vi "Migrate Shared Dependencies.vi"(0 "project path":path, 5 "measurement path":path, 7 "common dependencies":path[](array[path]), 11 "error in":errorcluster) -> (4 "outside items":string[](array[string]), 6 "library":T1[](array[typedef]), 15 "error out":errorcluster)   [LabVIEW 2021, in "Multiple Converter.lvlib"]
uses:
  Multiple Converter.lvlib
  TypeDefs/Library Info.ctl
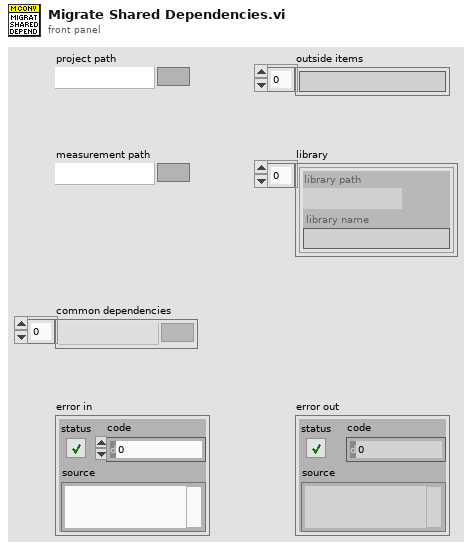
[diagram p1: front panel]
types:
  T1 = typedef "Multiple Converter.lvlib/Library Info.ctl" = cluster{"library path":path, "library name":string}
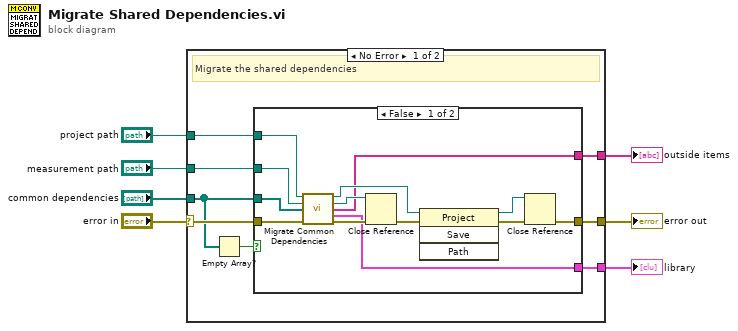
[diagram p0: block diagram]
diagram:
  n1 = case shown="No Error" "error in" {
    selector: "error in" -> [w14 w30]
    tunnel: [w15 w30] -> w7
    tunnel: "common dependencies" -> [w11 _]
    tunnel: "project path" -> [w13 _]
    tunnel: [w12 _] -> w3
    tunnel: "measurement path" -> [w9 _]
    tunnel: [w8 _] -> w1
    frame No Error {
      # "Migrate the shared dependencies"
      n2 = Empty Array?(array=w11) -> (empty?=w10:bool)
      n3 = case shown="False" w10 {
        tunnel: w14 -> [w28 w29]
        tunnel: [w24 w29] -> w15
        tunnel: w11 -> [w20 _]
        tunnel: w13 -> [w19 _]
        tunnel: [w18 _] -> w12
        tunnel: w9 -> [w17 _]
        tunnel: [w16 _] -> w8
        frame False {
          n4 = call "Migrate Common Dependencies.vi"("project path"=w19, "measurement path"=w17, "dependencies path"=w20, "error in"=w28) -> ("project reference"=w22:refnum<vi>, "measurement core reference"=w25:refnum<vi>, "outside items"=w18:string[], "library"=w16:T1[], "error out"=w27:errorcluster)  [unwired: 7 in]
          n5 = Close Reference(reference=w25, error in (no error)=w27) -> (error out=w26:errorcluster)
          n6 = invoke class="Project" method="Save"(reference=w22, error in=w26) -> (reference out=w21:refnum<vi>, error out=w23:errorcluster)  [unwired: 2 in, 2 out]
          n7 = Close Reference(reference=w21, error in (no error)=w23) -> (error out=w24:errorcluster)
        }
        frame True {
        }
      }
    }
    frame Error {
      # "Pass"
    }
  }
  "error out" <- w7
  "outside items" <- w3
  "library" <- w1
